vi "Get Descendants.vi"(8 "error in (no error)":errorcluster, 10 "Tag":string, 11 "Tree in":refnum<class "TreeControl.lvclass">) -> (0 "error out":errorcluster, 2 "DescendantTags[]":string[](array[string]), 3 "Tree out":refnum<class "TreeControl.lvclass">)   [LabVIEW 2015, in "TreeControl.lvclass"]
doc: "<b> </b> <b> </b>\n©2016 Q Software Innovations, LLC (QSI)\nwritten by Quentin Alldredge\nproduced in LabVIEW 2015\n\nsupport@qsoftwareinnovations.com\nwww.qsoftwareinnovations.com\n\nAll rights reserved.\n\nRedistribution and use in source and binary forms, with or without modification, are permitted provided that the following conditions are met:\n\n * Redistributions of source code must retain the above copyright notice, this list of conditions and the following disclaimer.\n * Redistributions in binary form must reproduce the above copyright notice, this list of conditions and the following disclaimer in the documentation and/or other materials provided with the distribution.\n * Neither the name of Q Software Innovations, LLC. nor the names of its contributors may be used to endorse or promote products derived from this software without specific prior written permission.\n\nTHIS SOFTWARE IS PROVIDED BY THE COPYRIGHT HOLDERS AND CONTRIBUTORS \"AS IS\" AND ANY EXPRESS OR IMPLIED WARRANTIES, INCLUDING, BUT NOT LIMITED TO, THE IMPLIED WARRANTIES OF MERCHANTABILITY AND FITNESS FOR A PARTICULAR PURPOSE ARE DISCLAIMED. IN NO EVENT SHALL THE COPYRIGHT OWNER OR CONTRIBUTORS BE LIABLE FOR ANY DIRECT, INDIRECT, INCIDENTAL, SPECIAL, EXEMPLARY, OR CONSEQUENTIAL DAMAGES (INCLUDING, BUT NOT LIMITED TO, PROCUREMENT OF SUBSTITUTE GOODS OR SERVICES; LOSS OF USE, DATA, OR PROFITS; OR BUSINESS INTERRUPTION) HOWEVER CAUSED AND ON ANY THEORY OF LIABILITY, WHETHER IN CONTRACT, STRICT LIABILITY, OR TORT (INCLUDING NEGLIGENCE OR OTHERWISE) ARISING IN ANY WAY OUT OF THE USE OF THIS SOFTWARE, EVEN IF ADVISED OF THE POSSIBILITY OF SUCH DAMAGE."
uses:
  TreeControl.lvclass
  TreeControl.lvclass/TreeControl.ctl
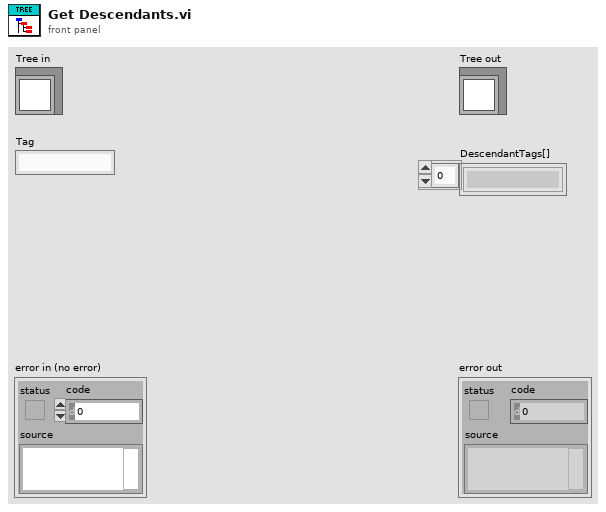
[diagram p1: front panel]
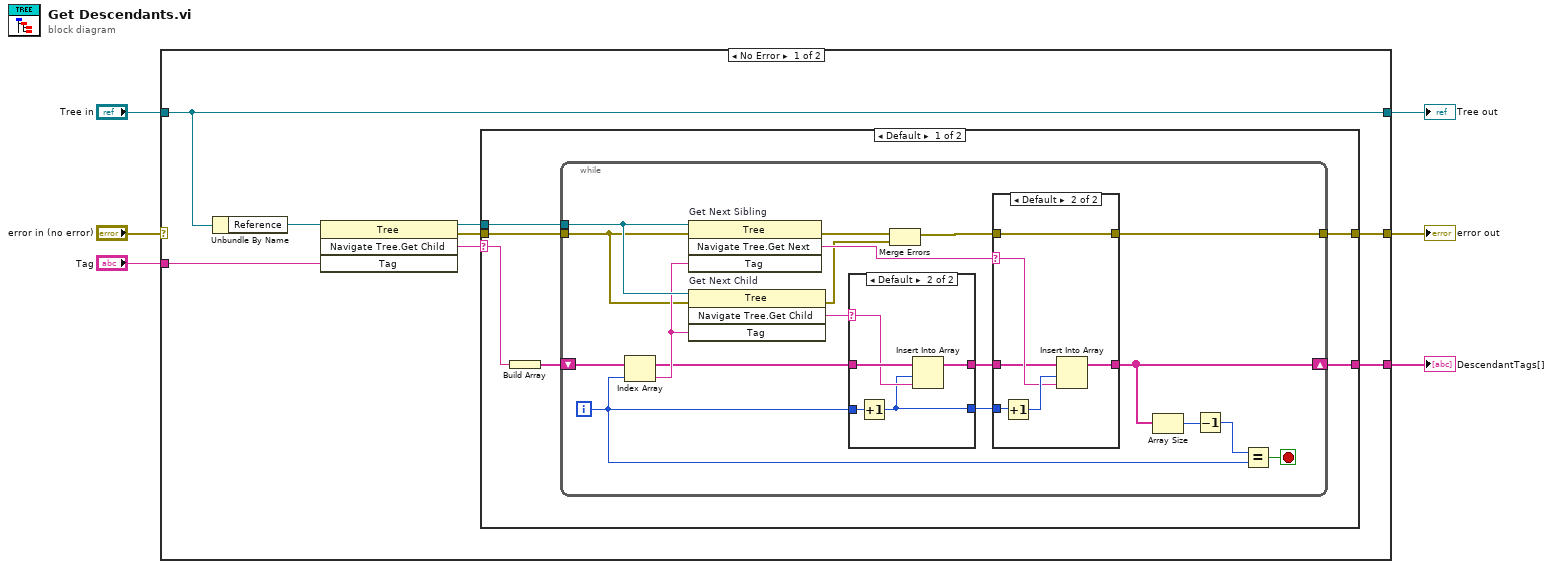
[diagram p0: block diagram]
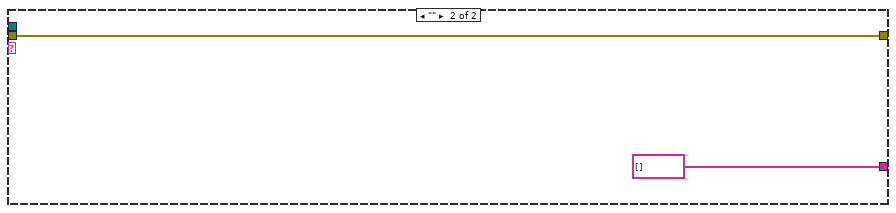
[diagram p4: hidden frame]
diagram:
  n1 = case shown="No Error" "error in (no error)" {
    selector: "error in (no error)" -> [_ w56]
    tunnel: [w10 w56] -> w5
    tunnel: [w8 w55] -> w3
    tunnel: "Tree in" -> [w8 w55]
    tunnel: "Tag" -> [w11 _]
    tunnel: [w9 _] -> w1
    frame No Error {
      n2 = Unbundle By Name(w8) -> ("Reference"=w7:refnum<vi>)
      n3 = invoke on="Invoke Node" class="Tree" method="Navigate Tree.Get Child"(reference=w7, "Tag"=w11) -> (reference out=w13:refnum<vi>, error out=w12:errorcluster, "Navigate Tree:Get Child"=w14:string)  [unwired: 2 in, 1 out]
      n4 = case shown="Default" w14 {
        selector: w14 -> [w16 _]
        tunnel: w13 -> [w20 _]
        tunnel: [w15 string[] []] -> w9
        tunnel: w12 -> [w19 w54]
        tunnel: [w17 w54] -> w10
        frame Default {
          n5 = Build Array(w16) -> (w18:string[])
          n6 = while {
            tunnel: w20 -> [w37]
            shift-right: [w30] -> w15
            shift-left: w18 -> [w35]
            tunnel: w19 -> [w23]
            tunnel: [w25] -> w17
            i -> [w26]
            stop <- w28 stop-if-true
            n7 = Index Array(array=w35, index=w26) -> (element=w36:string)
            n8 = invoke on="Get Next Sibling" class="Tree" method="Navigate Tree.Get Next"(reference=w37, error in=w23, "Tag"=w36) -> (error out=w24:errorcluster, "Navigate Tree:Get Next Item"=w33:string)  [unwired: 1 in, 2 out]
            n9 = invoke on="Get Next Child" class="Tree" method="Navigate Tree.Get Child"(reference=w37, error in=w23, "Tag"=w36) -> (error out=w21:errorcluster, "Navigate Tree:Get Child"=w34:string)  [unwired: 1 in, 2 out]
            n10 = case shown="Default" w34 {
              selector: w34 -> [_ w51]
              tunnel: w35 -> [w47 w52]
              tunnel: w26 -> [w46 w50]
              tunnel: [w47 w49] -> w31
              tunnel: [w46 w48] -> w32
              frame "" {
              }
              frame Default {
                n11 = Increment(x=w50) -> (x+1=w48:i32)
                n12 = Insert Into Array(array=w52, index=w48, new element=w51) -> (w49:string[])
              }
            }
            n13 = Merge Errors(w24, w21) -> (w22:errorcluster)
            n14 = case shown="Default" w33 {
              selector: w33 -> [_ w43]
              tunnel: w32 -> [_ w45]
              tunnel: w31 -> [w39 w42]
              tunnel: [w39 w41] -> w30
              tunnel: [w38 w40] -> w25
              tunnel: w22 -> [w38 w40]
              frame "" {
              }
              frame Default {
                n15 = Increment(x=w45) -> (x+1=w44:i32)
                n16 = Insert Into Array(array=w42, index=w44, new element=w43) -> (w41:string[])
              }
            }
            n17 = Array Size(array=w30) -> (size(s)=w29:i32)
            n18 = Decrement(x=w29) -> (x-1=w27:i32)
            n19 = Equal?(x=w27, y=w26) -> (x = y?=w28:bool)
          }
        }
        frame "" {
        }
      }
    }
    frame Error {
    }
  }
  "error out" <- w5
  "Tree out" <- w3
  "DescendantTags[]" <- w1
